vi "FormCalibra4.vi"() -> ()   [LabVIEW 2014]
uses:
  testMachine.ctl
  mainMachine.ctl
  <vilib>/Analysis/baseanly.llb/Mean (DBL).vi
  <vilib>/express/express shared/transition.llb/Dynamic To Waveform Array.vi
  <vilib>/express/express signal manip/GetorSetDDTAttributes/Set DDT Attributes/SetT0.vi
  <vilib>/express/express shared/transition.llb/Waveform Array To Dynamic.vi
  <vilib>/express/express signal manip/GetorSetDDTAttributes/Set DDT Attributes/Set DDT Properties.xnode
  <vilib>/Analysis/NI_AALBase.lvlib
panel:
  in  "editSetWaitTime":u32 caption="Tempo entre ciclos (ms)" max=999 step=1 format="%0d"
  in  "stop":bool
  out "ledSpeed":bool caption="Velocidade"
  out "error out":errorcluster
  out "ledAcquireState":bool caption="Acquire State"
  out "editTotalLowerLimit":dbl
  out "editCountLowerLimit":dbl
  out "editTotalUpperLimit":dbl
  out "editCountUpperLimit":dbl
  out "ledEnsaio 3":bool
  out "ledBrakeState":bool caption="Brake State"
  out "ledExitState":bool caption="Exit State"
  out "ledMotorState":bool caption="Motor State"
  out "ledInit2State":bool caption="Init State"
  out "ledBlockState":bool caption="Block State"
  out "ledRunningState":bool caption="Running State"
  out "ledReadyState":bool caption="Ready State"
  out "ledInitState":bool caption="Init State"
  out "mainMachine":T1
  out "testMachine":T2=enum."finish"
  in  "editSetPathToFile":path
  out "ledForce":bool caption="Célula de Carga"
  out "ledEngSpeed":bool caption="Rotação"
  out "ledTempB":bool caption="Temperatura B"
  out "ledTempA":bool caption="Temperatura A"
  out "ledTempRef":bool caption="Tempertura (Ref)"
  in  "buttonStop":bool
  in  "buttonStart":bool
  out "graphForce":dynamicdata(graph)
  in  "editOffsetForce":dbl caption="Tara" min=0.0 max=100.0 step=0.1
  in  "editSetForce":dbl caption="Fator de conversão"
  out "editForce":dbl caption="Força (Kgf)" format="%#_4f"
  out "graphSpeed":dynamicdata(graph)
  in  "editSetSpeed":dbl caption="Fator de conversão"
  out "editSpeed":dbl caption="Velocidade (km/h)" format="%#_4f"
  out "editEngineSpeed":dbl caption="Rotação (RPM)" format="%#_4f"
  in  "buttonMotor":bool
  in  "buttonBrake":bool
  in  "editSetWaitLowerTime":u32 caption="Tempo de espera (s)"
  in  "editSetWaitUpperTime":u32 caption="Tempo de espera (s)"
  in  "editSetNumberOfCycles":u32 caption="Número de ciclos" max=999 step=1 format="%0d"
  in  "editSetLowerLimit":u32 caption="Limite inferior (km/h)"
  in  "editSetUpperLimit":u32 caption="Limite superior (km/h)"
  out "editTempB":dbl caption="Temperatura B (ºC)"
  out "editTempA":dbl caption="Temperatura A (ºC)"
  in  "editSetTempRef":dbl caption="Offset referência" step=0.01 format="%#_2f"
  out "editTempRef":dbl caption="Referência (ºC)"
  out "ledMotor":bool
  out "ledBrake":bool
  out "ledEnsaio":bool
  out "labelTotalCycle":string
  out "labelCurrentCycle":string
  out "labelSystemTitle":string
  in  "editCurrCycleCtr":u32
  in  "velocidade 2":u32
  out "velocidade":u32
  # "Bancada de Frenagem - Ensaio"
  # "Sensores"
  # "Temperatura"
  # "Rotação"
  # "Célula de Carga"
  # "Configurações do ensaio"
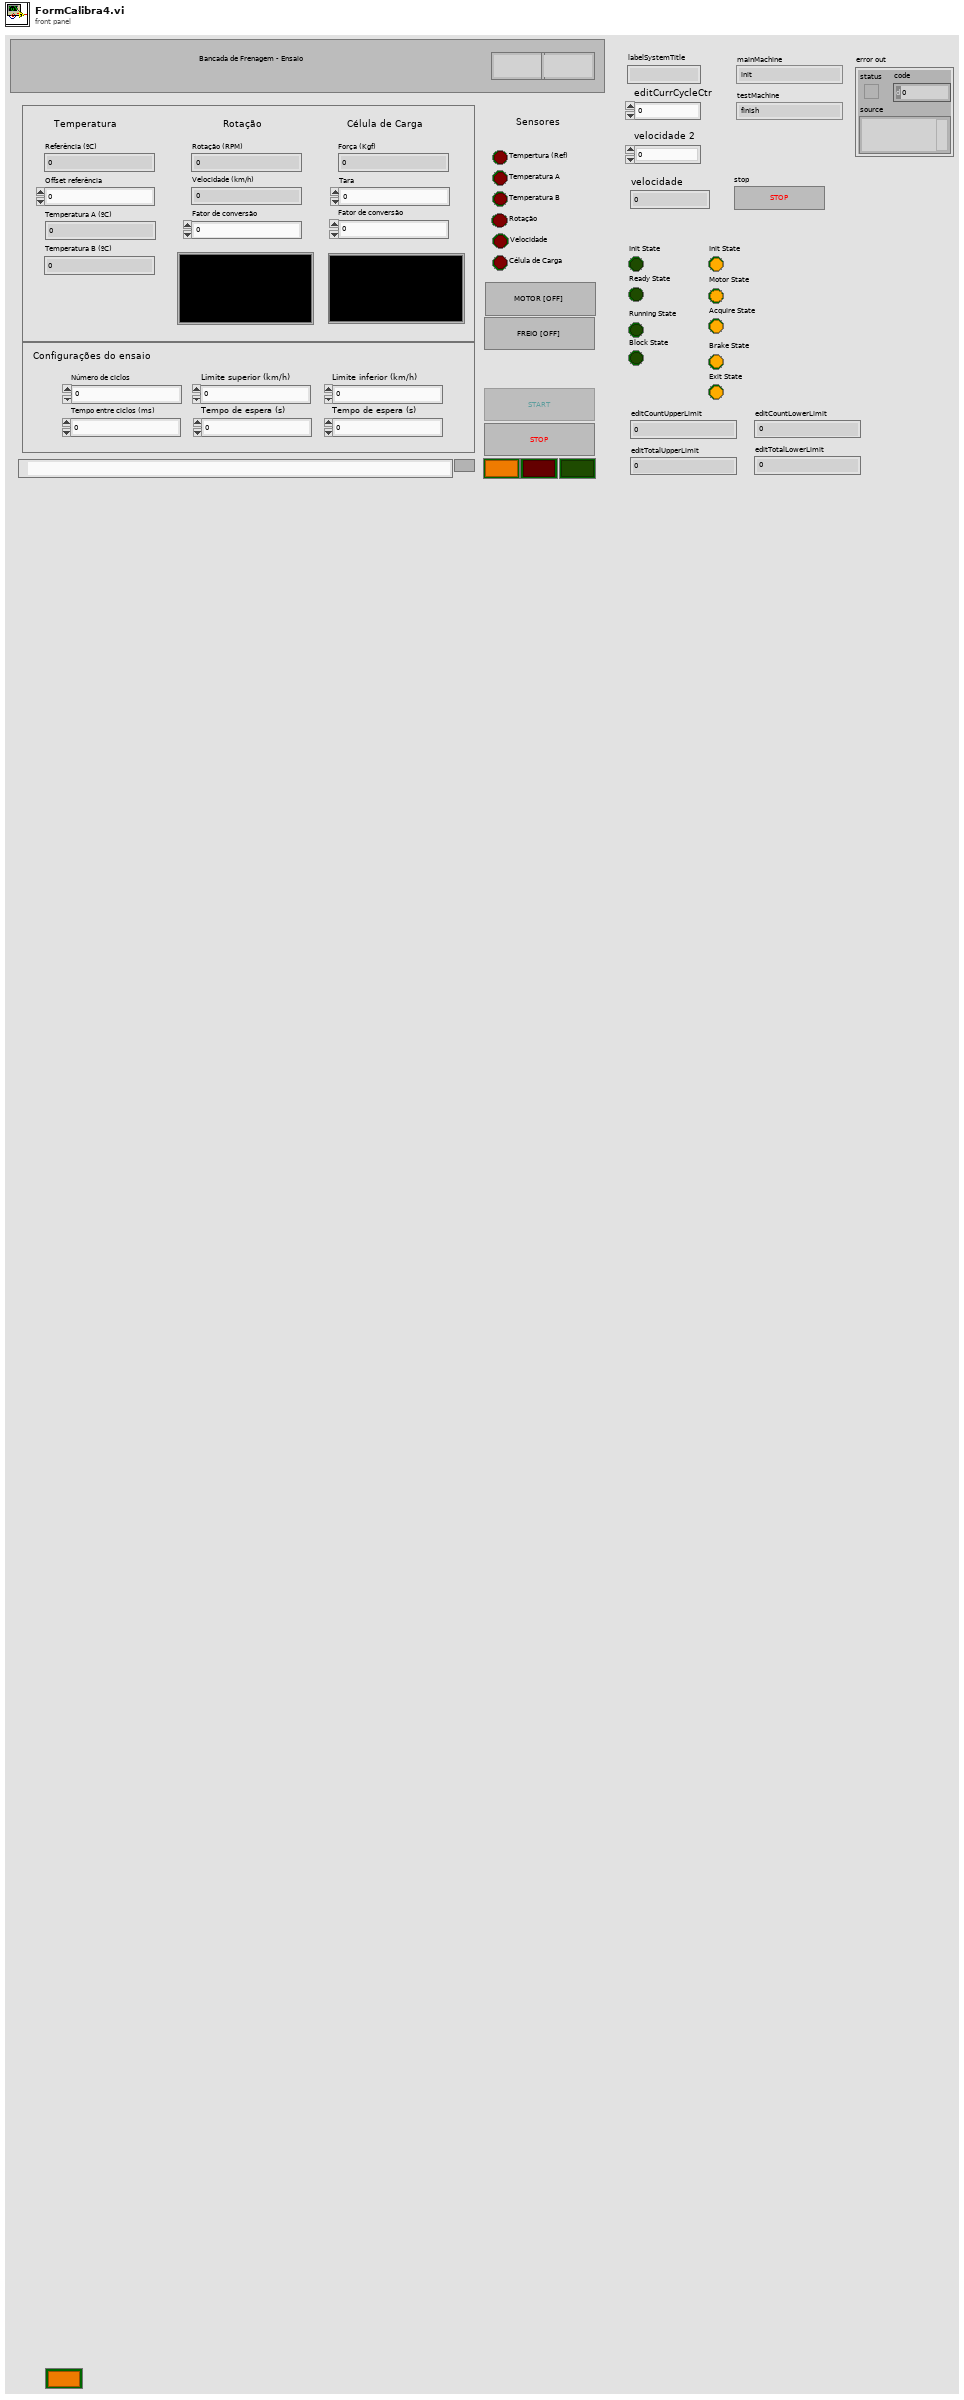
[diagram p1: front panel]
types:
  T1 = typedef "mainMachine.ctl" = enum16{"init", "ready", "running", "blocked", "finish"}
  T2 = typedef "testMachine.ctl" = enum16{"init", "motor", "motor acquire", "brake", "brake acquire", "wait ", "finish", "exit"}
  T3 = enum8{"Enabled", "Disabled", "Disabled and Grayed Out"}
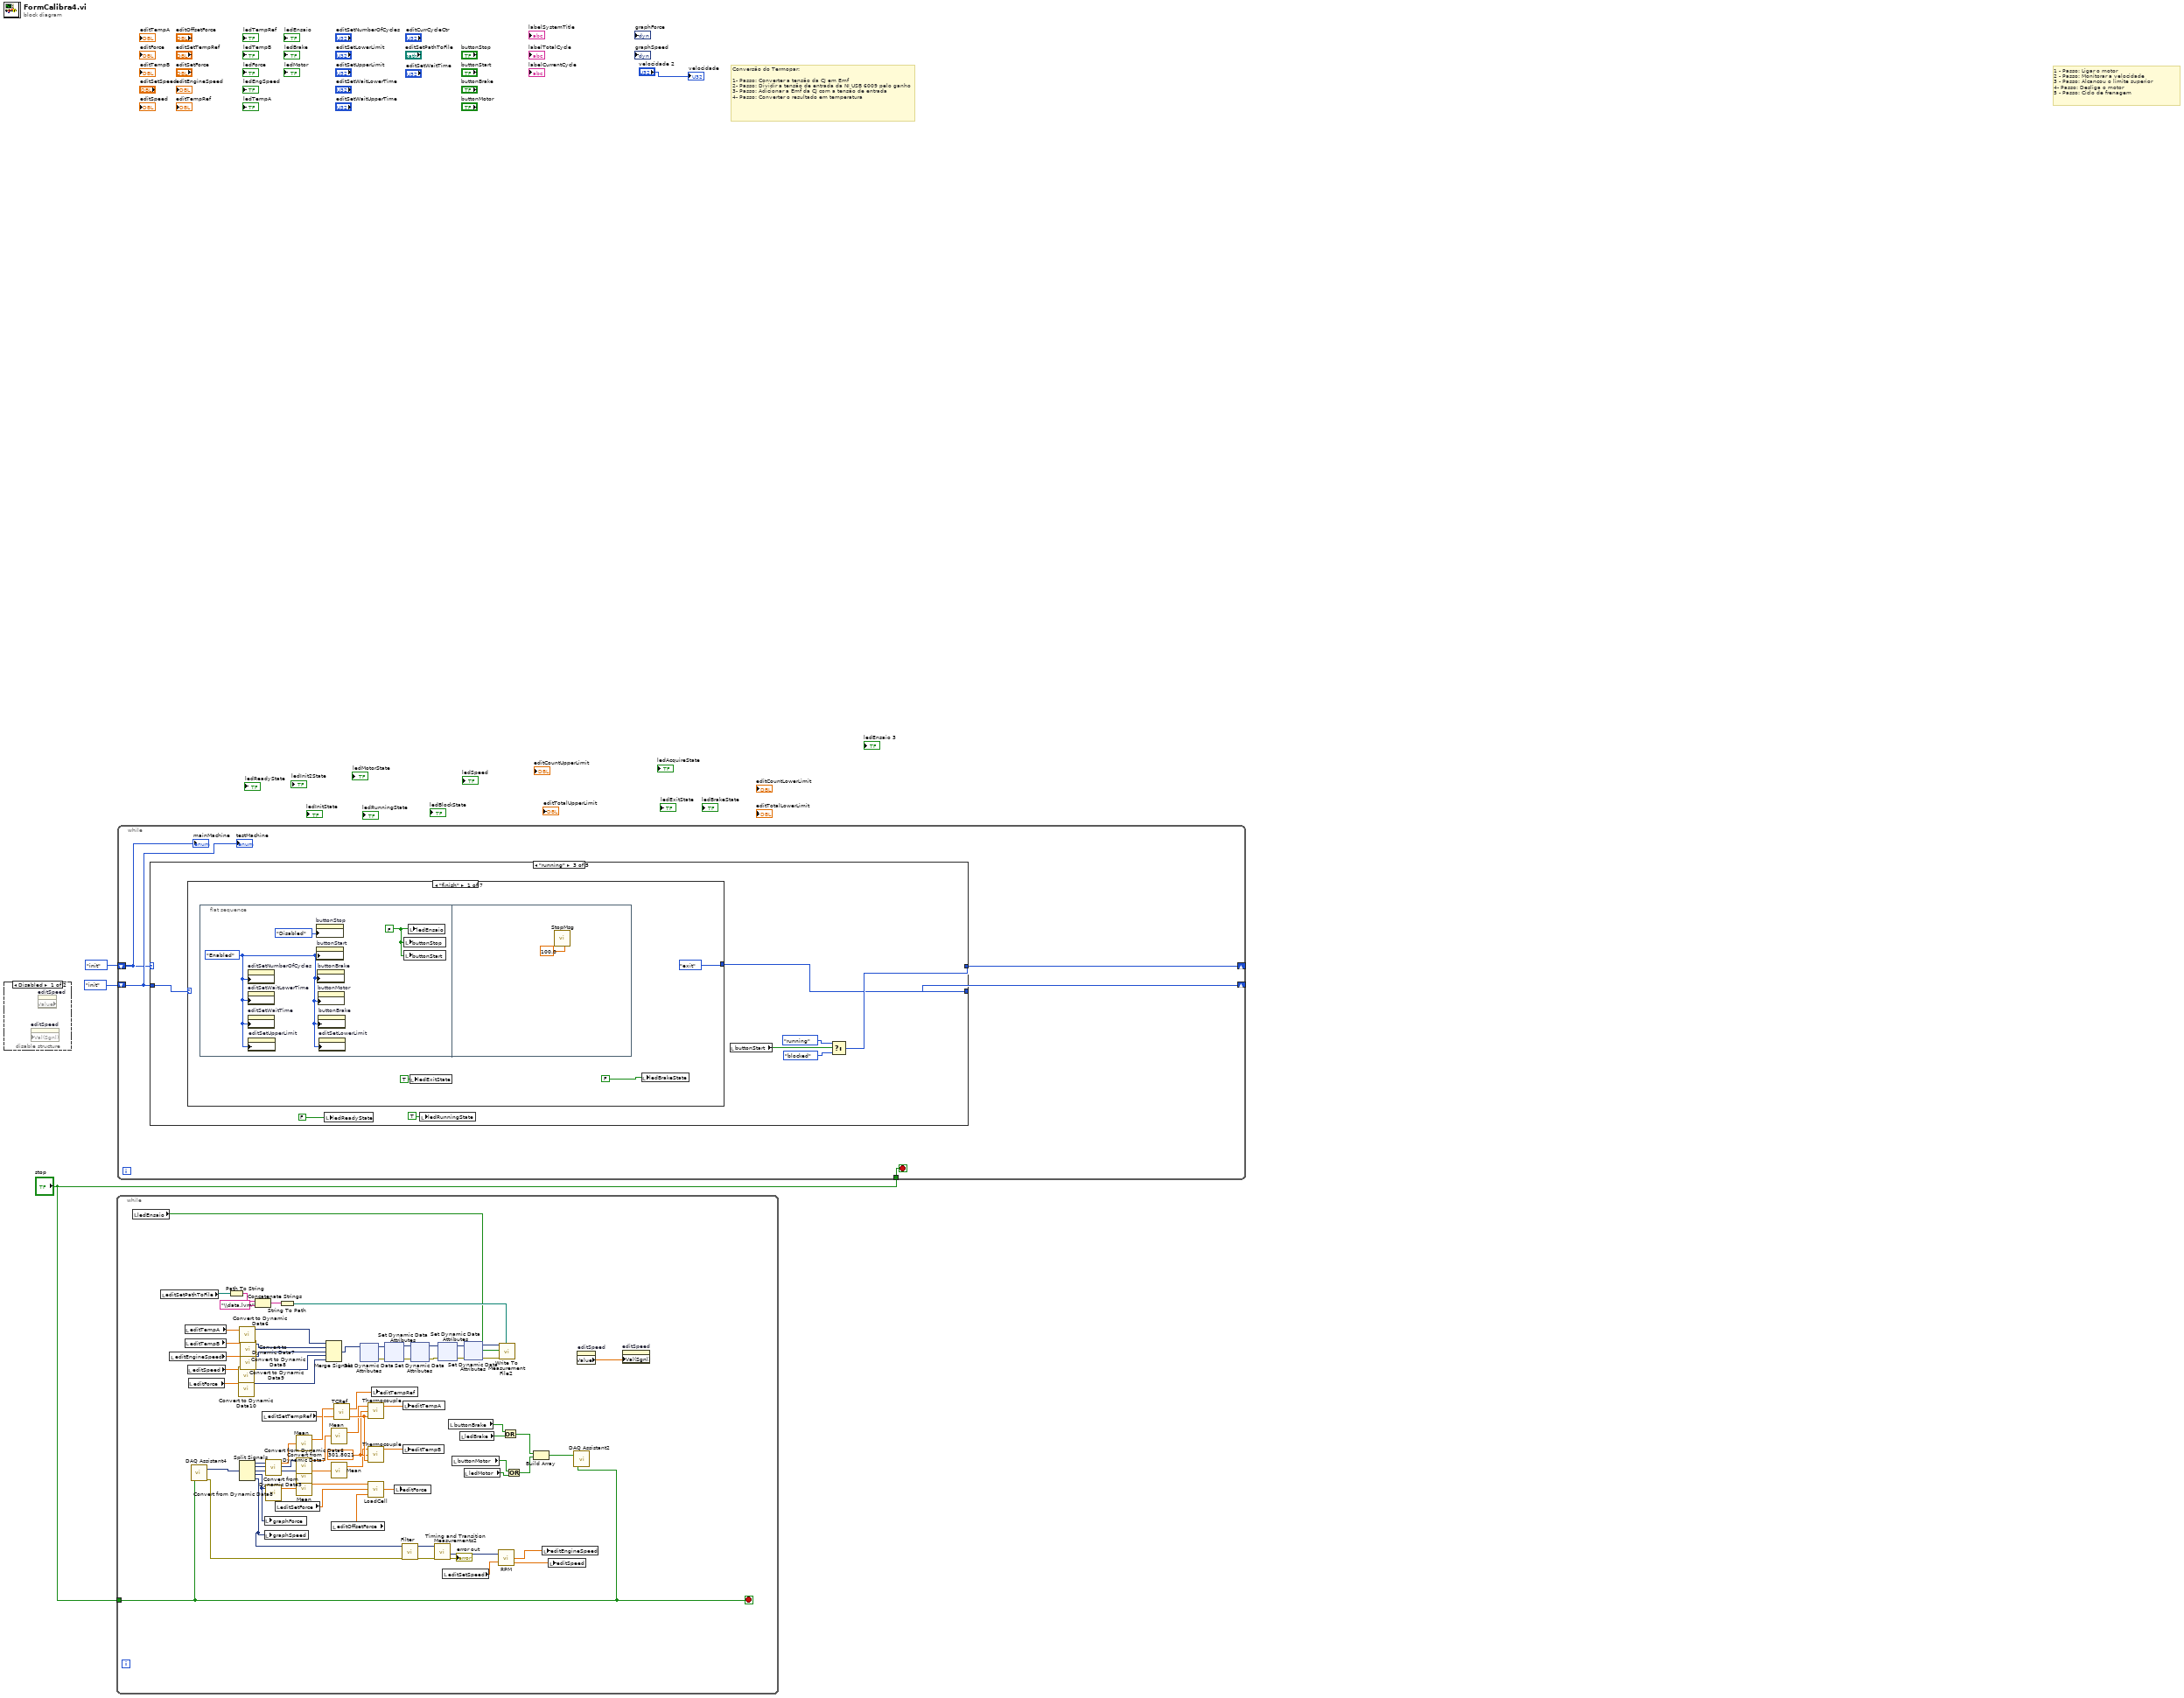
[diagram p0: block diagram]
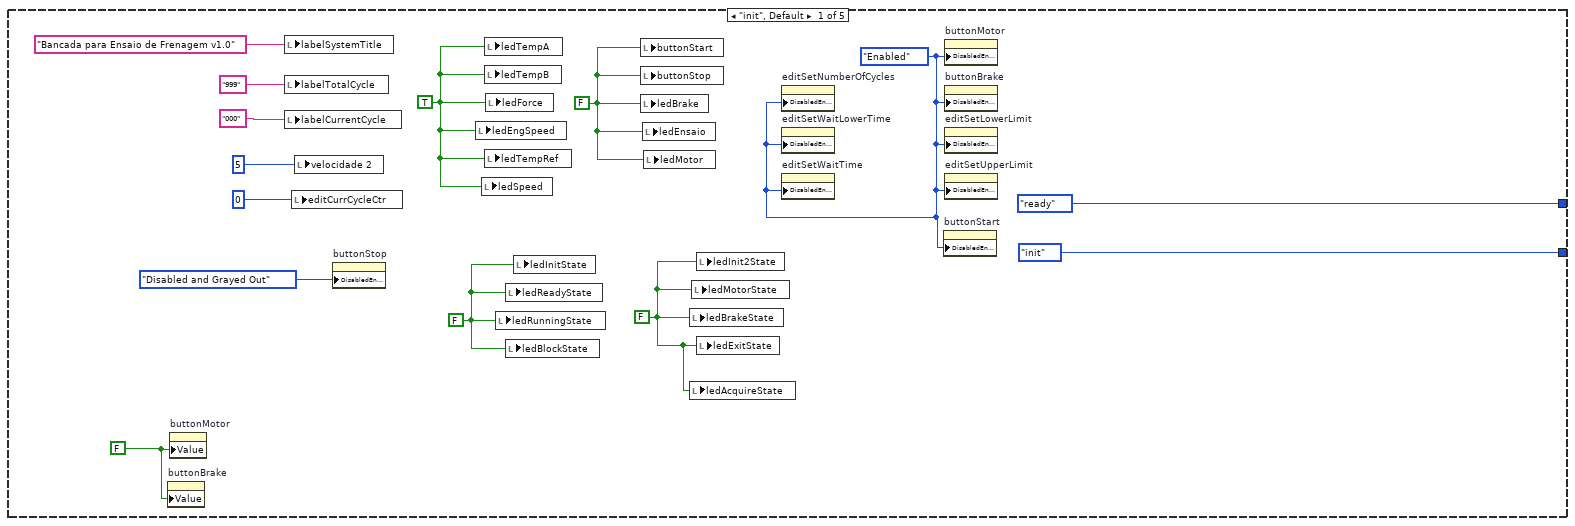
[diagram p3: hidden frame]
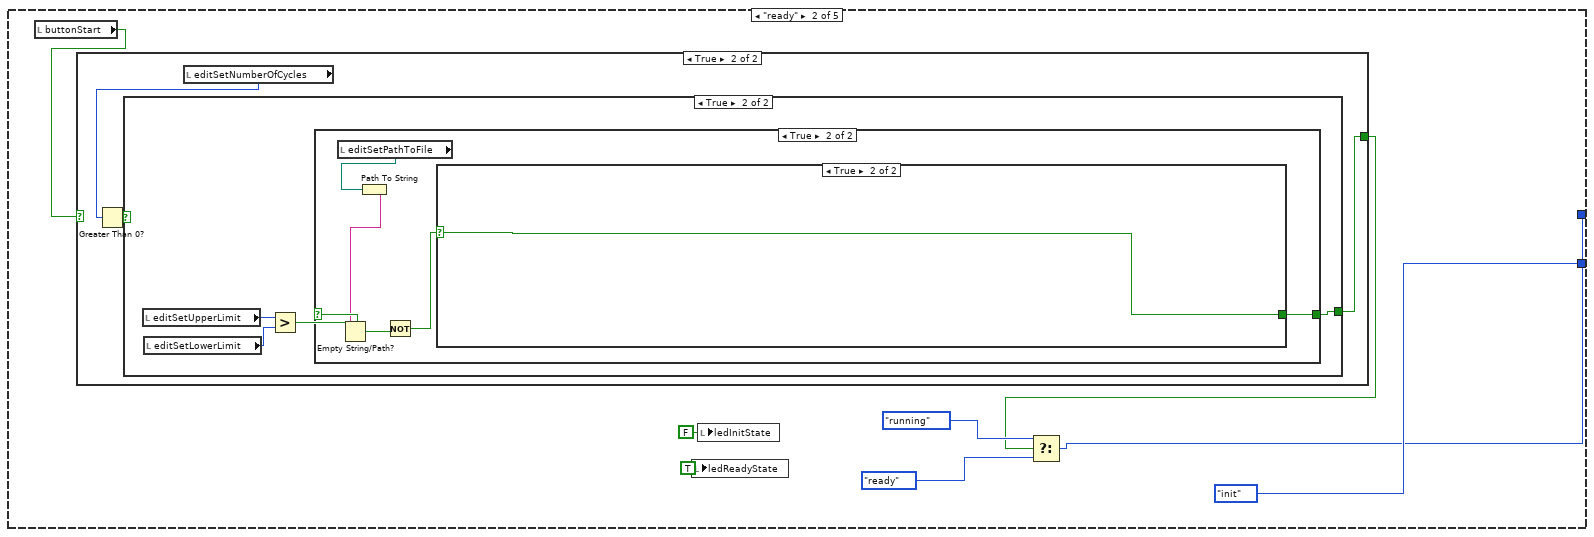
[diagram p4: hidden frame]
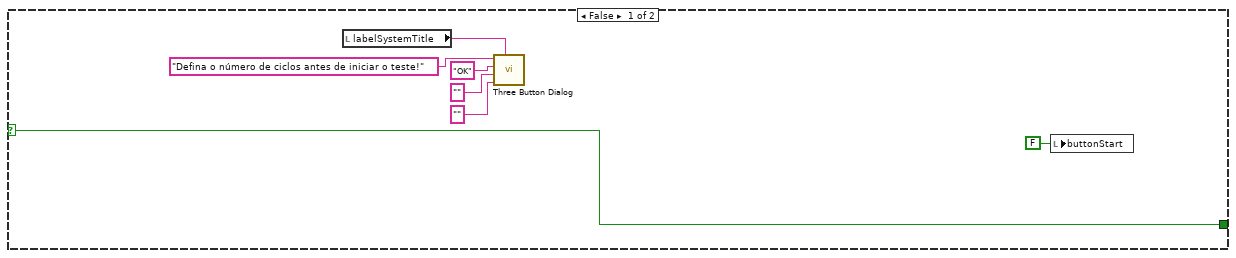
[diagram p6: hidden frame]
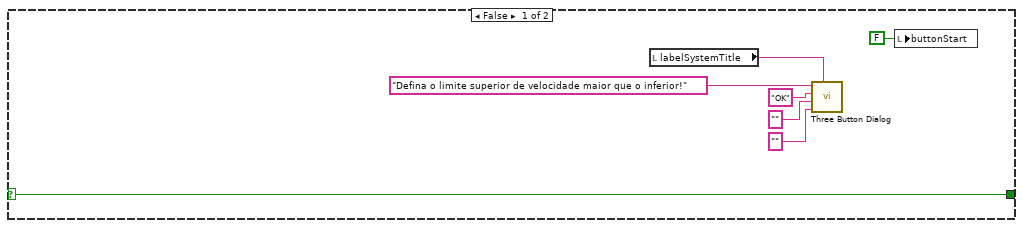
[diagram p7: hidden frame]
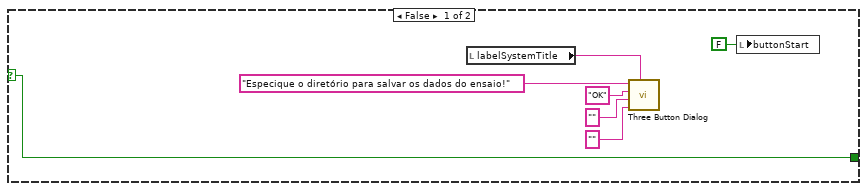
[diagram p8: hidden frame]
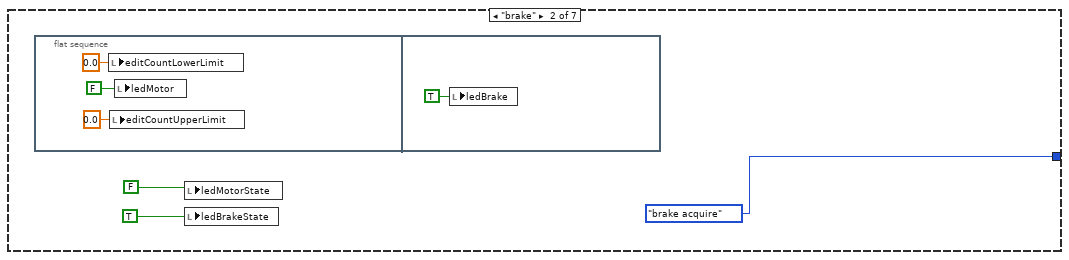
[diagram p9: hidden frame]
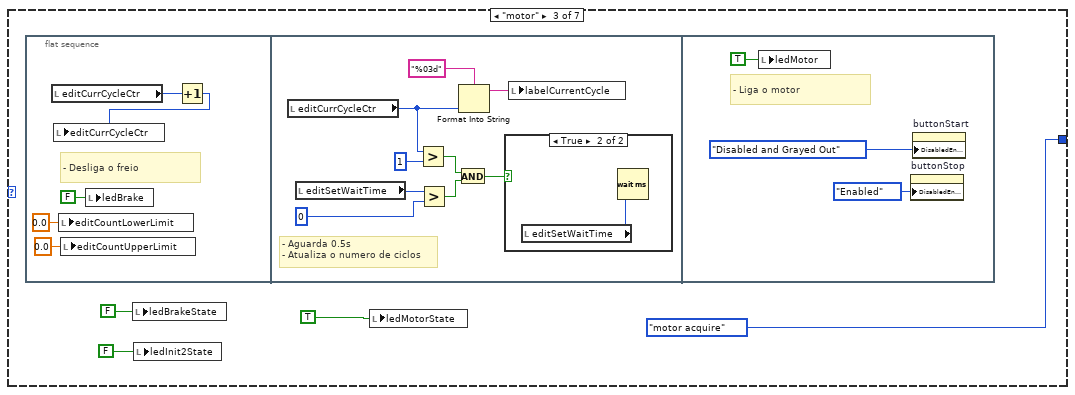
[diagram p10: hidden frame]
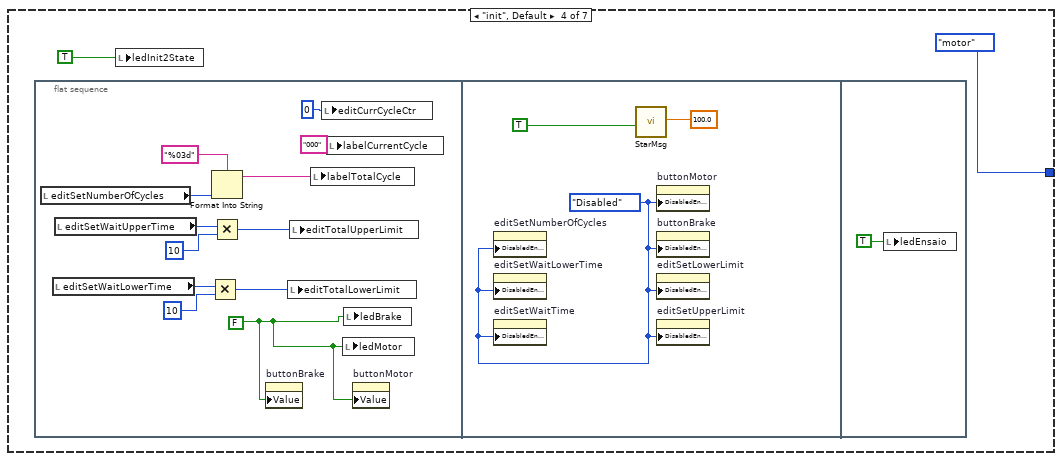
[diagram p12: hidden frame]
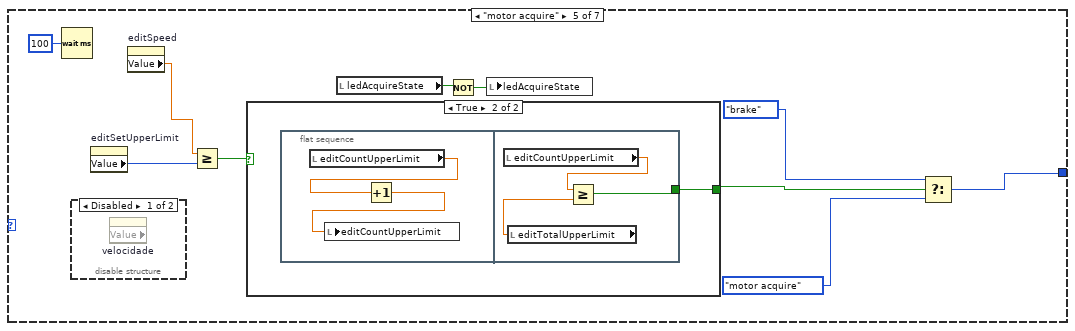
[diagram p13: hidden frame]
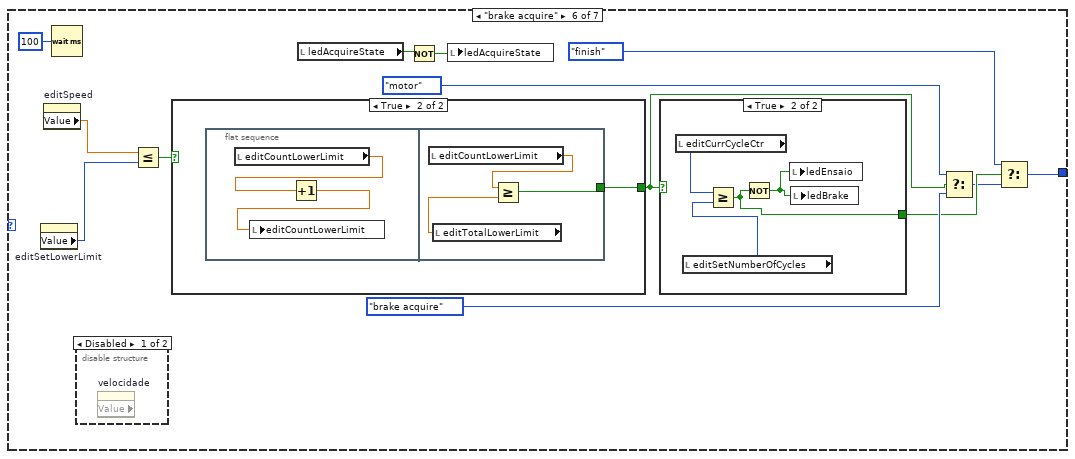
[diagram p16: hidden frame]
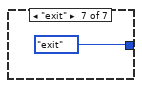
[diagram p20: hidden frame]
diagram:
  # "1 - Passo: Ligar o motor\n2 - Passo: Monitorar a velocidade\n3 - Passo: Alcancou o limite superior\n4- Passo: Desliga o motor\n5 - Passo: Ciclo de frenagem"
  # "Conversão do Termopar:\n\n1- Passo: Converter a tensão da CJ em Emf\n2- Passo: Dividir a tensão de entrada da NI USB 6009 pelo ganho\n3- Passo: Adicionar a Emf da CJ com a tensão de entrada\n4- Passo: Converter o resultado em temperatura"
  n1 = disable-structure shown="Disabled" {
    frame Disabled {
      n2 = property on="editSpeed" class="DigNum (strict)" props=["Val(Sgnl)"]() -> ()  [unwired: 3 in, 2 out]
      n3 = property on="editSpeed" class="DigNum (strict)" props=["Value"]() -> ()  [unwired: 2 in, 3 out]
    }
    frame Enabled {
    }
  }
  n4 = while {
    tunnel: "stop" -> [w5]
    stop <- w5 stop-if-true
    w31 = 301.8021 ("factor")
    n5 = local read "ledEnsaio"() -> (w6:bool)
    n6 = local read "editSetPathToFile"() -> (w47:path)
    n7 = local read "editEngineSpeed"() -> (w62:dbl)
    n8 = local read "editTempA"() -> (w59:dbl)
    n9 = local read "editTempB"() -> (w61:dbl)
    n10 = local read "editSpeed"() -> (w63:dbl)
    n11 = local read "editForce"() -> (w64:dbl)
    n12 = call "DAQ Assistant4"("stop (F)"=w5) -> ("data"=w20:dynamicdata, "error out"=w17:errorcluster)  [unwired: 15 in, 2 out]
    n13 = Path To String(path=w47) -> (string=w46:string)
    n14 = call "Convert to Dynamic Data9"("Double"=w63) -> ("Dynamic Data Type"=w67:dynamicdata)  [unwired: 3 in]
    n15 = call "Convert to Dynamic Data10"("Double"=w64) -> ("Dynamic Data Type"=w68:dynamicdata)  [unwired: 3 in]
    n16 = Split Signals(w20) -> (w23:dynamicdata, w27:dynamicdata, w25:dynamicdata, w36:dynamicdata, w16:dynamicdata)  [unwired: 5 in]
    n17 = call "Convert to Dynamic Data6"("Double"=w59) -> ("Dynamic Data Type"=w60:dynamicdata)  [unwired: 3 in]
    n18 = call "Convert to Dynamic Data7"("Double"=w61) -> ("Dynamic Data Type"=w65:dynamicdata)  [unwired: 3 in]
    n19 = call "Convert to Dynamic Data8"("Double"=w62) -> ("Dynamic Data Type"=w66:dynamicdata)  [unwired: 3 in]
    n20 = Concatenate Strings(w46, "\\data.lvm" ("string")) -> (w49:string)
    n21 = local read "editSetTempRef"() -> (w22:dbl)
    n22 = local write "graphForce"(w36) -> ()
    n23 = local write "graphSpeed"(w16) -> ()
    n24 = call "Convert from Dynamic Data5"("Dynamic Data Type"=w23) -> ("Array"=w44:dbl[])  [unwired: 3 in]
    n25 = call "Convert from Dynamic Data8"("Dynamic Data Type"=w36) -> ("Array"=w28:dbl[])  [unwired: 3 in]
    n26 = local read "editSetForce"() -> (w42:dbl)
    n27 = String To Path(string=w49) -> (path=w50:path)
    n28 = call-poly <vilib>:"Mean.vi"("X"=w44) -> ("mean"=w45:dbl)  [unwired: 1 out]
    n29 = call "Convert from Dynamic Data6"("Dynamic Data Type"=w27) -> ("Array"=w24:dbl[])  [unwired: 3 in]
    n30 = call "Convert from Dynamic Data7"("Dynamic Data Type"=w25) -> ("Array"=w26:dbl[])  [unwired: 3 in]
    n31 = call-poly <vilib>:"Mean.vi"("X"=w28) -> ("mean"=w35:dbl)  [unwired: 1 out]
    n32 = Merge Signals(w60, w65, w66, w67, w68) -> (w69:dynamicdata)
    n33 = call-poly <vilib>:"Mean.vi"("X"=w24) -> ("mean"=w29:dbl)  [unwired: 1 out]
    n34 = call-poly <vilib>:"Mean.vi"("X"=w26) -> ("mean"=w30:dbl)  [unwired: 1 out]
    n35 = local read "editOffsetForce"() -> (w43:dbl)
    n36 = call "TCRef.vi"("offset"=w22, "data"=w45) -> ("emf(mV)"=w32:dbl, "temp (degC)"=w21:dbl)
    n37 = xnode ("Set Dynamic Data Attributes")("Signals In"=w69) -> ("Signals Out"=w51:dynamicdata, "error out"=w53:errorcluster)  [unwired: 4 in]
    n38 = call "Thermocouple.vi"("cj(mV)"=w32, "factor"=w31, "data"=w29) -> ("temp(degC)"=w33:dbl)  [unwired: 2 out]
    n39 = call "Thermocouple.vi"("cj(mV)"=w32, "factor"=w31, "data"=w30) -> ("temp(degC)"=w34:dbl)  [unwired: 2 out]
    n40 = call "LoadCell.vi"("tara"=w43, "factor"=w42, "data"=w35) -> ("force (Kgf)"=w39:dbl)
    n41 = local write "editTempRef"(w21) -> ()
    n42 = xnode ("Set Dynamic Data Attributes")("Signals In"=w51, "error in"=w53) -> ("Signals Out"=w52:dynamicdata, "error out"=w54:errorcluster)  [unwired: 3 in]
    n43 = local write "editForce"(w39) -> ()
    n44 = call "Filter"("error in (no error)"=w17, "Signal"=w16) -> ("error out"=w18:errorcluster, "Filtered Signal"=w15:dynamicdata)  [unwired: 8 in]
    n45 = local write "editTempA"(w33) -> ()
    n46 = local write "editTempB"(w34) -> ()
    n47 = xnode ("Set Dynamic Data Attributes")("Signals In"=w52, "error in"=w54) -> ("Signals Out"=w70:dynamicdata, "error out"=w55:errorcluster)  [unwired: 3 in]
    n48 = call "Timing and Transition Measurements2"("error in (no error)"=w18, "Signals"=w15) -> ("error out"=→"error out":errorcluster, "Frequency"=w37:dynamicdata)  [unwired: 8 in]
    n49 = xnode ("Set Dynamic Data Attributes")("Signals In"=w70, "error in"=w55) -> ("Signals Out"=w71:dynamicdata, "error out"=w56:errorcluster)  [unwired: 3 in]
    n50 = local read "editSetSpeed"() -> (w38:dbl)
    n51 = local read "buttonBrake"() -> (w10:bool)
    n52 = local read "buttonMotor"() -> (w12:bool)
    n53 = local read "ledBrake"() -> (w8:bool)
    n54 = xnode ("Set Dynamic Data Attributes")("Signals In"=w71, "error in"=w56) -> ("Signals Out"=w57:dynamicdata, "error out"=w58:errorcluster)  [unwired: 3 in]
    n55 = local read "ledMotor"() -> (w11:bool)
    n56 = call "RPM.vi"("data"=w37, "factor"=w38) -> ("RPM"=w40:dbl, "km/h"=w41:dbl)  [unwired: 1 out]
    n57 = call "Write To Measurement File2"("Signals"=w57, "Enable"=w6, "error in (no error)"=w58, "Filename"=w50) -> ()  [unwired: 13 in, 3 out]
    n58 = Or(x=w10, y=w8) -> (x .or. y?=w9:bool)
    n59 = Or(x=w12, y=w11) -> (x .or. y?=w13:bool)
    n60 = Build Array(w9, w13) -> (w7:bool[])
    n61 = local write "editEngineSpeed"(w40) -> ()
    n62 = local write "editSpeed"(w41) -> ()
    n63 = call "DAQ Assistant2"("data"=w7, "stop (T)"=w5) -> ()  [unwired: 16 in, 2 out]
    n64 = property on="editSpeed" class="DigNum (strict)"() -> ("Value"=w14:dbl)  [unwired: 2 in, 2 out]
    n65 = property on="editSpeed" class="DigNum (strict)"("Val(Sgnl)"=w14) -> ()  [unwired: 2 in, 2 out]
  }
  n66 = while {
    shift-right: [w166] -> _
    shift-left: mainMachine."init" ("mainMachine") -> [w163]
    shift-right: [w165] -> _
    shift-left: testMachine."init" ("testMachine") -> [w164]
    tunnel: "stop" -> [w162]
    stop <- w162 stop-if-true
    n67 = case shown="\"running\"" w163 {
      tunnel: [mainMachine."ready" ("mainMachine") w181 w226 w329 mainMachine."finish" ("mainMachine")] -> w166
      tunnel: [testMachine."init" ("testMachine") testMachine."init" ("testMachine") w225 testMachine."init" ("testMachine") testMachine."init" ("testMachine")] -> w165
      tunnel: w164 -> [_ _ w224 _ _]
      frame "init", Default {
        w167 = T3."Enabled" ("Disabled")
        w169 = FALSE ("buttonMotor")
        w172 = FALSE
        w173 = FALSE
        w168 = TRUE
        w177 = FALSE ("motor")
        n68 = property on="buttonBrake" class="Bool (strict)"("Value"=w169) -> ()  [unwired: 2 in, 2 out]
        n69 = property on="buttonMotor" class="Bool (strict)"("Value"=w169) -> ()  [unwired: 2 in, 2 out]
        n70 = local write "labelSystemTitle"("Bancada para Ensaio de Frenagem v1.0" ("systemTitle")) -> ()
        n71 = local write "labelTotalCycle"("999" ("totalCycle")) -> ()
        n72 = local write "labelCurrentCycle"("000" ("currentCycle")) -> ()
        n73 = local write "editCurrCycleCtr"(u32 0 ("currentCycleCtr")) -> ()
        n74 = local write "velocidade 2"(u32 5 ("velocidade 2")) -> ()
        n75 = property on="buttonStop" class="Bool (strict)"("DisabledEnum"=T3."Disabled and Grayed Out" ("Disabled")) -> ()  [unwired: 2 in, 2 out]
        n76 = local write "ledEngSpeed"(w168) -> ()
        n77 = local write "ledSpeed"(w168) -> ()
        n78 = local write "ledTempA"(w168) -> ()
        n79 = local write "ledTempB"(w168) -> ()
        n80 = local write "ledTempRef"(w168) -> ()
        n81 = local write "ledForce"(w168) -> ()
        n82 = local write "ledRunningState"(w173) -> ()
        n83 = local write "ledReadyState"(w173) -> ()
        n84 = local write "ledBlockState"(w173) -> ()
        n85 = local write "ledInitState"(w173) -> ()
        n86 = local write "buttonStart"(w177) -> ()
        n87 = local write "buttonStop"(w177) -> ()
        n88 = local write "ledBrake"(w177) -> ()
        n89 = local write "ledEnsaio"(w177) -> ()
        n90 = local write "ledMotor"(w177) -> ()
        n91 = local write "ledBrakeState"(w172) -> ()
        n92 = local write "ledAcquireState"(w172) -> ()
        n93 = local write "ledMotorState"(w172) -> ()
        n94 = local write "ledInit2State"(w172) -> ()
        n95 = local write "ledExitState"(w172) -> ()
        n96 = property on="editSetNumberOfCycles" class="DigNum (strict)"("DisabledEnum"=w167) -> ()  [unwired: 2 in, 2 out]
        n97 = property on="editSetWaitLowerTime" class="DigNum (strict)"("DisabledEnum"=w167) -> ()  [unwired: 2 in, 2 out]
        n98 = property on="editSetWaitTime" class="DigNum (strict)"("DisabledEnum"=w167) -> ()  [unwired: 2 in, 2 out]
        n99 = property on="buttonStart" class="Bool (strict)"("DisabledEnum"=w167) -> ()  [unwired: 2 in, 2 out]
        n100 = property on="buttonMotor" class="Bool (strict)"("DisabledEnum"=w167) -> ()  [unwired: 2 in, 2 out]
        n101 = property on="buttonBrake" class="Bool (strict)"("DisabledEnum"=w167) -> ()  [unwired: 2 in, 2 out]
        n102 = property on="editSetLowerLimit" class="DigNum (strict)"("DisabledEnum"=w167) -> ()  [unwired: 2 in, 2 out]
        n103 = property on="editSetUpperLimit" class="DigNum (strict)"("DisabledEnum"=w167) -> ()  [unwired: 2 in, 2 out]
      }
      frame "ready" {
        n104 = local read "buttonStart"() -> (w184:bool)
        n105 = case shown="True" w184 {
          selector: w184 -> [w189 _]
          tunnel: [w189 w190] -> w183
          frame False {
          }
          frame True {
            n106 = local read "editSetNumberOfCycles"() -> (w191:u32)
            n107 = Greater Than 0?(x=w191) -> (x > 0?=w192:bool)
            n108 = case shown="True" w192 {
              selector: w192 -> [w199 _]
              tunnel: [w199 w200] -> w190
              frame False {
                n109 = local read "labelSystemTitle"() -> (w194:string)
                n110 = call <vilib>:"Three Button Dialog.vi"("Window Title (\"\")"=w194, "Right Button Text (\"Cancel\")"="" ("Right Button Text (\"Cancel\")"), "Center Button Text (\"No\")"="" ("Center Button Text (\"No\")"), "Left Button Text (\"Yes\")"="OK" ("Left Button Text (\"Yes\")"), "message"="Defina o número de ciclos antes de iniciar o teste!") -> ()  [unwired: 6 in, 1 out]
                n111 = local write "buttonStart"(FALSE ("startButton")) -> ()
              }
              frame True {
                n112 = local read "editSetUpperLimit"() -> (w202:u32)
                n113 = local read "editSetLowerLimit"() -> (w201:u32)
                n114 = Greater?(x=w202, y=w201) -> (0:w203:bool)
                n115 = case shown="True" w203 {
                  selector: w203 -> [w210 _]
                  tunnel: [w210 w213] -> w200
                  frame False {
                    n116 = local read "labelSystemTitle"() -> (w205:string)
                    n117 = call <vilib>:"Three Button Dialog.vi"("Window Title (\"\")"=w205, "Right Button Text (\"Cancel\")"="" ("Right Button Text (\"Cancel\")"), "Center Button Text (\"No\")"="" ("Center Button Text (\"No\")"), "Left Button Text (\"Yes\")"="OK" ("Left Button Text (\"Yes\")"), "message"="Defina o limite superior de velocidade maior que o inferior!") -> ()  [unwired: 6 in, 1 out]
                    n118 = local write "buttonStart"(FALSE ("startButton")) -> ()
                  }
                  frame True {
                    n119 = local read "editSetPathToFile"() -> (w215:path)
                    n120 = Path To String(path=w215) -> (string=w214:string)
                    n121 = Empty String/Path?(string/path=w214) -> (empty?=w212:bool)
                    n122 = Not(x=w212) -> (.not. x?=w211:bool)
                    n123 = case shown="True" w211 {
                      selector: w211 -> [w222 w223]
                      tunnel: [w222 w223] -> w213
                      frame False {
                        n124 = local read "labelSystemTitle"() -> (w217:string)
                        n125 = call <vilib>:"Three Button Dialog.vi"("Window Title (\"\")"=w217, "Right Button Text (\"Cancel\")"="" ("Right Button Text (\"Cancel\")"), "Center Button Text (\"No\")"="" ("Center Button Text (\"No\")"), "Left Button Text (\"Yes\")"="OK" ("Left Button Text (\"Yes\")"), "message"="Especique o diretório para salvar os dados do ensaio!") -> ()  [unwired: 6 in, 1 out]
                        n126 = local write "buttonStart"(FALSE ("startButton")) -> ()
                      }
                      frame True {
                      }
                    }
                  }
                }
              }
            }
          }
        }
        n127 = local write "ledReadyState"(TRUE ("ledReady")) -> ()
        n128 = local write "ledInitState"(FALSE ("ledReady")) -> ()
        n129 = Select(t=mainMachine."running" ("mainMachine"), s=w183, f=mainMachine."ready" ("mainMachine")) -> (s? t:f=w181:T1)
      }
      frame "running" {
        n130 = case shown="\"finish\"" w224 {
          tunnel: [testMachine."exit" ("testMachine") testMachine."brake acquire" ("testMachine") testMachine."motor acquire" ("testMachine") testMachine."motor" ("testMachine") w287 w308 testMachine."exit" ("testMachine")] -> w225
          frame "finish" {
            n131 = flat-sequence {
              frame #0 {
                w236 = FALSE ("ledReady")
                w235 = T3."Enabled" ("Disabled")
                n132 = property on="editSetNumberOfCycles" class="DigNum (strict)"("DisabledEnum"=w235) -> ()  [unwired: 2 in, 2 out]
                n133 = property on="editSetWaitLowerTime" class="DigNum (strict)"("DisabledEnum"=w235) -> ()  [unwired: 2 in, 2 out]
                n134 = property on="editSetWaitTime" class="DigNum (strict)"("DisabledEnum"=w235) -> ()  [unwired: 2 in, 2 out]
                n135 = property on="editSetUpperLimit" class="DigNum (strict)"("DisabledEnum"=w235) -> ()  [unwired: 2 in, 2 out]
                n136 = property on="buttonStop" class="Bool (strict)"("DisabledEnum"=T3."Disabled" ("Disabled")) -> ()  [unwired: 2 in, 2 out]
                n137 = property on="buttonStart" class="Bool (strict)"("DisabledEnum"=w235) -> ()  [unwired: 2 in, 2 out]
                n138 = property on="buttonBrake" class="Bool (strict)"("DisabledEnum"=w235) -> ()  [unwired: 2 in, 2 out]
                n139 = property on="buttonMotor" class="Bool (strict)"("DisabledEnum"=w235) -> ()  [unwired: 2 in, 2 out]
                n140 = property on="buttonBrake" class="Bool (strict)"("DisabledEnum"=w235) -> ()  [unwired: 2 in, 2 out]
                n141 = property on="editSetLowerLimit" class="DigNum (strict)"("DisabledEnum"=w235) -> ()  [unwired: 2 in, 2 out]
                n142 = local write "buttonStop"(w236) -> ()
                n143 = local write "buttonStart"(w236) -> ()
                n144 = local write "ledEnsaio"(w236) -> ()
              }
              frame #1 {
                n145 = call "StopMsg.vi"("Max Value (100)"=100.0) -> ()  [unwired: 8 in, 2 out]
              }
            }
            n146 = local write "ledExitState"(TRUE ("ledReady")) -> ()
            n147 = local write "ledBrakeState"(FALSE ("ledReady")) -> ()
          }
          frame "brake" {
            n148 = flat-sequence {
              frame #0 {
                n149 = local write "editCountLowerLimit"(0.0 ("editCountUpperLimit")) -> ()
                n150 = local write "editCountUpperLimit"(0.0 ("editCountUpperLimit")) -> ()
                n151 = local write "ledMotor"(FALSE ("motor")) -> ()
              }
              frame #1 {
                n152 = local write "ledBrake"(TRUE ("freio")) -> ()
              }
            }
            n153 = local write "ledMotorState"(FALSE ("ledReady")) -> ()
            n154 = local write "ledBrakeState"(TRUE ("ledReady")) -> ()
          }
          frame "motor" {
            n155 = flat-sequence {
              frame #0 {
                # "- Desliga o freio"
                n156 = local read "editCurrCycleCtr"() -> (w253:u32)
                n157 = local write "editCountLowerLimit"(0.0 ("editCountUpperLimit")) -> ()
                n158 = local write "editCountUpperLimit"(0.0 ("editCountUpperLimit")) -> ()
                n159 = local write "ledBrake"(FALSE ("freio")) -> ()
                n160 = Increment(x=w253) -> (x+1=w252:u32)
                n161 = local write "editCurrCycleCtr"(w252) -> ()
              }
              frame #1 {
                # "- Aguarda 0.5s \n- Atualiza o numero de ciclos"
                n162 = local read "editCurrCycleCtr"() -> (w259:u32)
                n163 = local read "editSetWaitTime"() -> (w261:u32)
                n164 = Greater?(x=w259, y=u32 1) -> (0:w256:bool)
                n165 = Greater?(x=w261, y=u32 0) -> (0:w255:bool)
                n166 = And(x=w256, y=w255) -> (x .and. y?=w257:bool)
                n167 = Format Into String(format string="%03d", w259) -> (resulting string=w262:string)  [unwired: 2 in, 1 out]
                n168 = case shown="True" w257 {
                  frame False {
                  }
                  frame True {
                    n169 = local read "editSetWaitTime"() -> (w264:u32)
                    n170 = Wait (ms)(milliseconds to wait=w264) -> ()  [unwired: 1 out]
                  }
                }
                n171 = local write "labelCurrentCycle"(w262) -> ()
              }
              frame #2 {
                # "- Liga o motor"
                n172 = local write "ledMotor"(TRUE ("motor")) -> ()
                n173 = property on="buttonStop" class="Bool (strict)"("DisabledEnum"=T3."Enabled" ("Disabled")) -> ()  [unwired: 2 in, 2 out]
                n174 = property on="buttonStart" class="Bool (strict)"("DisabledEnum"=T3."Disabled and Grayed Out" ("Disabled")) -> ()  [unwired: 2 in, 2 out]
              }
            }
            n175 = local write "ledBrakeState"(FALSE ("ledReady")) -> ()
            n176 = local write "ledInit2State"(FALSE ("ledReady")) -> ()
            n177 = local write "ledMotorState"(TRUE ("ledReady")) -> ()
          }
          frame "init", Default {
            n178 = flat-sequence {
              frame #0 {
                w270 = FALSE ("ensaio")
                n179 = local read "editSetNumberOfCycles"() -> (w279:u32)
                n180 = local read "editSetWaitLowerTime"() -> (w271:u32)
                n181 = local read "editSetWaitUpperTime"() -> (w276:u32)
                n182 = Multiply(x=w271, y=u32 10) -> (x*y=w273:u32)
                n183 = Format Into String(format string="%03d", w279) -> (resulting string=w280:string)  [unwired: 2 in, 1 out]
                n184 = Multiply(x=w276, y=u32 10) -> (x*y=w274:u32)
                n185 = property on="buttonBrake" class="Bool (strict)"("Value"=w270) -> ()  [unwired: 2 in, 2 out]
                n186 = local write "editTotalLowerLimit"(w273) -> ()
                n187 = local write "editTotalUpperLimit"(w274) -> ()
                n188 = local write "labelTotalCycle"(w280) -> ()
                n189 = local write "editCurrCycleCtr"(u32 0 ("currentCycleCtr")) -> ()
                n190 = local write "labelCurrentCycle"("000" ("currentCycle")) -> ()
                n191 = local write "ledMotor"(w270) -> ()
                n192 = local write "ledBrake"(w270) -> ()
                n193 = property on="buttonMotor" class="Bool (strict)"("Value"=w270) -> ()  [unwired: 2 in, 2 out]
              }
              frame #1 {
                w282 = T3."Disabled" ("Disabled")
                n194 = property on="editSetNumberOfCycles" class="DigNum (strict)"("DisabledEnum"=w282) -> ()  [unwired: 2 in, 2 out]
                n195 = property on="editSetWaitLowerTime" class="DigNum (strict)"("DisabledEnum"=w282) -> ()  [unwired: 2 in, 2 out]
                n196 = property on="editSetWaitTime" class="DigNum (strict)"("DisabledEnum"=w282) -> ()  [unwired: 2 in, 2 out]
                n197 = call "StarMsg.vi"("Show"=TRUE, "Max Value (100)"=100.0) -> ()  [unwired: 7 in, 2 out]
                n198 = property on="buttonMotor" class="Bool (strict)"("DisabledEnum"=w282) -> ()  [unwired: 2 in, 2 out]
                n199 = property on="buttonBrake" class="Bool (strict)"("DisabledEnum"=w282) -> ()  [unwired: 2 in, 2 out]
                n200 = property on="editSetLowerLimit" class="DigNum (strict)"("DisabledEnum"=w282) -> ()  [unwired: 2 in, 2 out]
                n201 = property on="editSetUpperLimit" class="DigNum (strict)"("DisabledEnum"=w282) -> ()  [unwired: 2 in, 2 out]
              }
              frame #2 {
                n202 = local write "ledEnsaio"(TRUE ("ensaio")) -> ()
              }
            }
            n203 = local write "ledInit2State"(TRUE ("ledReady")) -> ()
          }
          frame "motor acquire" {
            n204 = Wait (ms)(milliseconds to wait=u32 100) -> ()  [unwired: 1 out]
            n205 = disable-structure shown="Disabled" {
              frame Disabled {
                n206 = property on="velocidade" class="DigNum (strict)" props=["Value"]() -> ()  [unwired: 2 in, 3 out]
              }
              frame Enabled {
              }
            }
            n207 = property on="editSetUpperLimit" class="DigNum (strict)"() -> ("Value"=w294:u32)  [unwired: 2 in, 2 out]
            n208 = property on="editSpeed" class="DigNum (strict)"() -> ("Value"=w286:dbl)  [unwired: 2 in, 2 out]
            n209 = Greater Or Equal?(x=w286, y=w294) -> (x >= y?=w291:bool)
            n210 = case shown="True" w291 {
              selector: w291 -> [w296 _]
              tunnel: [w296 w297] -> w290
              frame False {
              }
              frame True {
                n211 = flat-sequence {
                  tunnel: [w300] -> w297
                  frame #0 {
                    n212 = local read "editCountUpperLimit"() -> (w298:dbl)
                    n213 = Increment(x=w298) -> (x+1=w299:dbl)
                    n214 = local write "editCountUpperLimit"(w299) -> ()
                  }
                  frame #1 {
                    n215 = local read "editCountUpperLimit"() -> (w302:dbl)
                    n216 = local read "editTotalUpperLimit"() -> (w301:dbl)
                    n217 = Greater Or Equal?(x=w302, y=w301) -> (x >= y?=w300:bool)
                  }
                }
              }
            }
            n218 = local read "ledAcquireState"() -> (w293:bool)
            n219 = Not(x=w293) -> (.not. x?=w292:bool)
            n220 = local write "ledAcquireState"(w292) -> ()
            n221 = Select(t=testMachine."brake" ("testMachine"), s=w290, f=testMachine."motor acquire" ("testMachine")) -> (s? t:f=w287:T2)
          }
          frame "brake acquire" {
            n222 = property on="editSetLowerLimit" class="DigNum (strict)"() -> ("Value"=w307:u32)  [unwired: 2 in, 2 out]
            n223 = property on="editSpeed" class="DigNum (strict)"() -> ("Value"=w303:dbl)  [unwired: 2 in, 2 out]
            n224 = Wait (ms)(milliseconds to wait=u32 100) -> ()  [unwired: 1 out]
            n225 = disable-structure shown="Disabled" {
              frame Disabled {
                n226 = property on="velocidade" class="DigNum (strict)" props=["Value"]() -> ()  [unwired: 2 in, 3 out]
              }
              frame Enabled {
              }
            }
            n227 = Less Or Equal?(x=w303, y=w307) -> (x <= y?=w312:bool)
            n228 = case shown="True" w312 {
              selector: w312 -> [w321 _]
              tunnel: [w321 w322] -> w310
              frame False {
              }
              frame True {
                n229 = flat-sequence {
                  tunnel: [w325] -> w322
                  frame #0 {
                    n230 = local read "editCountLowerLimit"() -> (w323:dbl)
                    n231 = Increment(x=w323) -> (x+1=w324:dbl)
                    n232 = local write "editCountLowerLimit"(w324) -> ()
                  }
                  frame #1 {
                    n233 = local read "editCountLowerLimit"() -> (w327:dbl)
                    n234 = local read "editTotalLowerLimit"() -> (w326:dbl)
                    n235 = Greater Or Equal?(x=w327, y=w326) -> (x >= y?=w325:bool)
                  }
                }
              }
            }
            n236 = local read "ledAcquireState"() -> (w314:bool)
            n237 = Not(x=w314) -> (.not. x?=w313:bool)
            n238 = local write "ledAcquireState"(w313) -> ()
            n239 = case shown="True" w310 {
              selector: w310 -> [w316 _]
              tunnel: [w316 w318] -> w306
              frame False {
              }
              frame True {
                n240 = local read "editCurrCycleCtr"() -> (w319:u32)
                n241 = local read "editSetNumberOfCycles"() -> (w320:u32)
                n242 = Greater Or Equal?(x=w319, y=w320) -> (x >= y?=w318:bool)
                n243 = Not(x=w318) -> (.not. x?=w317:bool)
                n244 = local write "ledEnsaio"(w317) -> ()
                n245 = local write "ledBrake"(w317) -> ()
              }
            }
            n246 = Select(t=testMachine."motor" ("testMachine"), s=w310, f=testMachine."brake acquire" ("testMachine")) -> (s? t:f=w305:T2)
            n247 = Select(t=testMachine."finish" ("testMachine"), s=w306, f=w305) -> (s? t:f=w308:T2)
          }
          frame "exit" {
          }
        }
        n248 = local write "ledReadyState"(FALSE ("ledReady")) -> ()
        n249 = local write "ledRunningState"(TRUE ("ledReady")) -> ()
        n250 = local read "buttonStart"() -> (w229:bool)
        n251 = Select(t=mainMachine."running" ("mainMachine"), s=w229, f=mainMachine."blocked" ("mainMachine")) -> (s? t:f=w226:T1)
      }
      frame "blocked" {
        n252 = local read "buttonStart"() -> (w333:bool)
        n253 = Select(t=mainMachine."ready" ("mainMachine"), s=w333, f=mainMachine."blocked" ("mainMachine")) -> (s? t:f=w329:T1)
        n254 = local write "ledRunningState"(FALSE ("ledReady")) -> ()
        n255 = local write "ledBlockState"(TRUE ("ledReady")) -> ()
      }
      frame "finish" {
        n256 = local write "ledBlockState"(FALSE ("ledReady")) -> ()
      }
    }
    "mainMachine" <- w163
    "testMachine" <- w164
  }
  "velocidade" <- "velocidade 2"
